vi "Periodic Tasks.vi"(8 "error in":errorcluster) -> ()   [LabVIEW 2014]
doc: "This VI runs in parallel to other tasks. It can contain as many user-defined periodic loops as you need. These can carry out PID or other sorts of timed response."
uses:
  Robot Global Data.vi
  <vilib>/Rock Robotics/Network Tables/SD Write Number.vi
  <vilib>/Rock Robotics/Network Tables/SD Write Numeric Array.vi
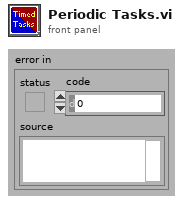
[diagram p1: front panel]
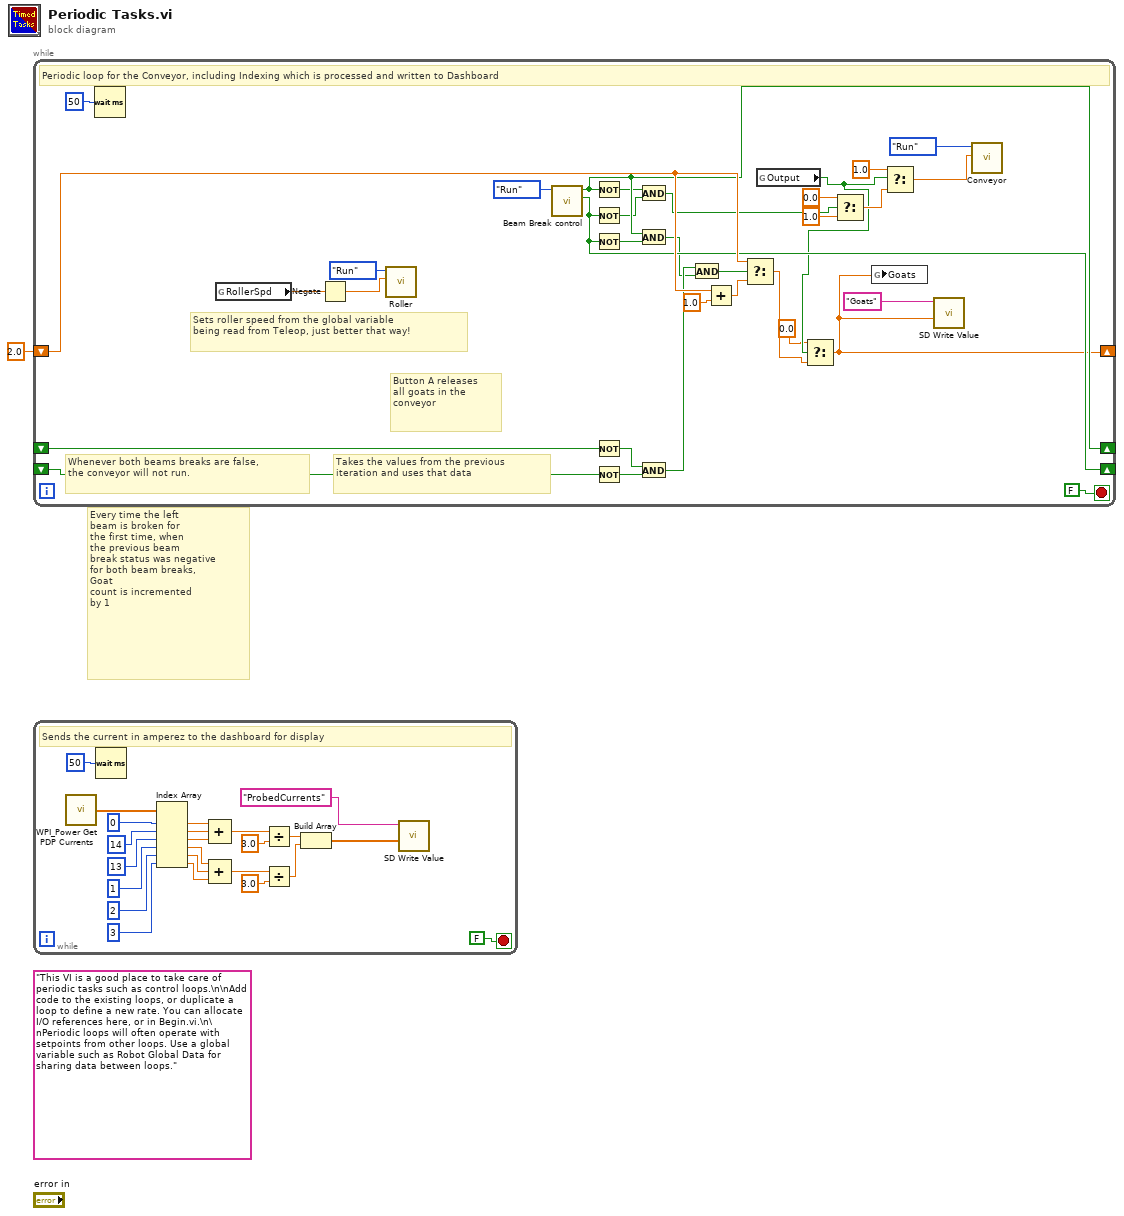
[diagram p0: block diagram]
diagram:
  (unwired) "This VI is a good place to take care of periodic tasks such as control loops.\n\nAdd code to the existing loops, or duplicate a loop to define a new rate. You can allocate I/O references here, or in Begin.vi.\n\nPeriodic loops will often operate with setpoints from other loops. Use a global variable such as Robot Global Data for sharing data between loops."
  # "Every time the left\nbeam is broken for\nthe first time, when\nthe previous beam\nbreak status was negative\nfor both beam breaks,\nGoat\ncount is incremented\nby 1"
  n1 = while {
    shift-right: [w15] -> _
    shift-left: 2.0 ("f") -> [w29]
    shift-right: [w25] -> _
    shift-left: _ -> [w20]
    shift-right: [w26] -> _
    shift-left: _ -> [w19]
    stop <- FALSE stop-if-true
    # "Sets roller speed from the global variable\nbeing read from Teleop, just better that way!"
    # "Takes the values from the previous\niteration and uses that data"
    # "Button A releases\nall goats in the \nconveyor"
    # "Whenever both beams breaks are false,\nthe conveyor will not run."
    # "Periodic loop for the Conveyor, including Indexing which is processed and written to Dashboard"
    n2 = Wait (ms)(milliseconds to wait=u32 50) -> ()  [unwired: 1 out]
    n3 = global read "Robot Global Data.vi" "RollerSpd"() -> (w5:dbl)
    n4 = Negate(x=w5) -> (-x=w2:dbl)
    n5 = call "Roller.vi"("RollerSpeed"=w2, "Enum"=enum16{"Start", "Run", "End"}."Run") -> ()  [unwired: 10 in]
    n6 = call "Beam Break control.vi"("SRE ENUM"=enum16{"Start", "Run", "End"}."Run") -> ("2nd BB"=w26:bool, "1st BB"=w25:bool)  [unwired: 9 in]
    n7 = Not(x=w25) -> (.not. x?=w24:bool)
    n8 = Not(x=w26) -> (.not. x?=w23:bool)
    n9 = Not(x=w26) -> (.not. x?=w27:bool)
    n10 = Not(x=w20) -> (.not. x?=w21:bool)
    n11 = Not(x=w19) -> (.not. x?=w22:bool)
    n12 = And(x=w24, y=w23) -> (x .and. y?=w9:bool)
    n13 = And(x=w25, y=w27) -> (x .and. y?=w17:bool)
    n14 = And(x=w21, y=w22) -> (x .and. y?=w18:bool)
    n15 = And(x=w18, y=w17) -> (x .and. y?=w16:bool)
    n16 = Add(x=w29, y=1.0) -> (x+y=w30:dbl)
    n17 = Select(t=w29, s=w16, f=w30) -> (s? t:f=w4:dbl)
    n18 = global read "Robot Global Data.vi" "Output"() -> (w7:bool)
    n19 = Select(t=0.0 ("f"), s=w7, f=w4) -> (s? t:f=w15:dbl)
    n20 = Select(t=0.0, s=w9, f=1.0) -> (s? t:f=w11:dbl)
    n21 = global write "Robot Global Data.vi" "Goats"(w15) -> ()
    n22 = Select(t=1.0, s=w7, f=w11) -> (s? t:f=w13:dbl)
    n23 = call-poly <vilib>:"SD Write Value.vi"("Numeric"=w15, "Name"="Goats") -> ()  [unwired: 8 in, 2 out]
    n24 = call "Conveyor.vi"("Speed"=w13, "Enum"=enum16{"Start", "Run", "End"}."Run") -> ()  [unwired: 10 in]
  }
  n25 = while {
    stop <- FALSE stop-if-true
    # "Sends the current in amperez to the dashboard for display"
    n26 = call <vilib>:"WPI_Power Get PDP Currents.vi"() -> ("all currents (A)"=w55:dbl[])  [unwired: 13 in, 2 out]
    n27 = Wait (ms)(milliseconds to wait=u32 50) -> ()  [unwired: 1 out]
    n28 = Index Array(array=w55, index #1=0 ("index"), index #2=14 ("index"), index #3=13 ("index"), index #4=1 ("index"), index #5=2 ("index"), index #6=3 ("index")) -> (element #1=w48:dbl, element #2=w47:dbl, element #3=w46:dbl, element #4=w41:dbl, element #5=w40:dbl, element #6=w39:dbl)
    n29 = Compound Arithmetic op=ADD(w48, w47, w46) -> (w42:dbl)
    n30 = Compound Arithmetic op=ADD(w41, w40, w39) -> (w43:dbl)
    n31 = Divide(x=w42, y=3.0) -> (x/y=w38:dbl)
    n32 = Divide(x=w43, y=3.0) -> (x/y=w37:dbl)
    n33 = Build Array(w38, w37) -> (w35:dbl[])
    n34 = call-poly <vilib>:"SD Write Value.vi"("Numeric Array"=w35, "Name"="ProbedCurrents") -> ()  [unwired: 8 in, 2 out]
  }
